vi "Keypad(subvi).vi"(6 "[ESC]":bool, 7 "DIO Ref Out 4":T1, 8 "error in (no error)":errorcluster, 9 "DIO Ref Out":T1, 10 "DIO Ref Out 2":T1, 11 "DIO Ref Out 3":T1) -> (0 "error out":errorcluster, 1 "Array":T8, 2 "Scan":bool[](array[boolean]), 3 "Index of current pressed button":i32)   [LabVIEW 2017]
uses:
  tranparent_key.ctl
  <vilib>/myRIO/Instrument Drivers/Onboard IO/DIO/typedefs/DIO Reference.ctl
  <vilib>/myRIO/Common/Instrument Driver Framework/Utilities/typedefs/myRIO Generic Hardware Reference.ctl
  <vilib>/myRIO/Common/Instrument Driver Framework/Utilities/typedefs/Hardware Version Enum.ctl
  <vilib>/myRIO/Common/Instrument Driver Framework/Utilities/typedefs/myRIO v1.0 Reference.ctl
  <vilib>/myRIO/Common/Instrument Driver Framework/Utilities/typedefs/Generic FPGA Reference.ctl
  <vilib>/myRIO/Common/Instrument Driver Framework/myRIO v1.0/DIO/typedefs/DIO Channels List.ctl
  <vilib>/myRIO/Common/Instrument Driver Framework/myRIO v1.0/DIO/typedefs/DIO Channels Enum.ctl
  <vilib>/Utility/error.llb/Error Cluster From Error Code.vi
  <vilib>/myRIO/Common/Instrument Driver Framework/myRIO v1.0/DIO/vis/myRIO v1.0 Read DIO.vi
  <vilib>/myRIO/Common/Instrument Driver Framework/myRIO v1.0/DIO/vis/myRIO v1.0 Write DIO.vi
  <vilib>/myRIO/Instrument Drivers/Onboard IO/DIO/vis/Smart Open.vi
  <vilib>/myRIO/Instrument Drivers/Onboard IO/DIO/DIO.lvlib
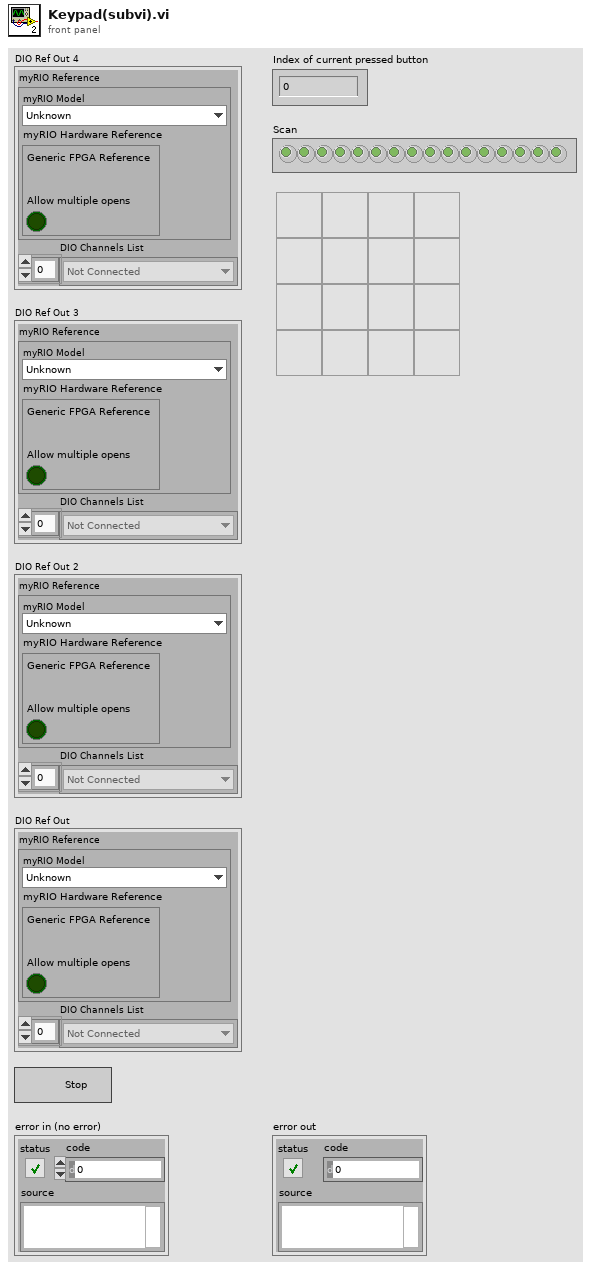
[diagram p1: front panel]
types:
  T1 = typedef "DIO.lvlib/DIO Reference.ctl" = cluster{"myRIO Reference":T2, "DIO Channels List":T6}
  T2 = typedef "myRIO Generic Hardware Reference.ctl" = cluster{"myRIO Model":T3, "myRIO Hardware Reference":T4}
  T3 = typedef "Hardware Version Enum.ctl" = enum16{"Unknown", "myRIO-1900", "myRIO-1950", "roboRIO", "NI ELVIS RIO CM"}
  T4 = typedef "myRIO v1.0 Reference.ctl" = cluster{"Generic FPGA Reference":T5, "Allow multiple opens":bool}
  T5 = typedef "Generic FPGA Reference.ctl" = refnum<k20>
  T6 = typedef "DIO Channels List.ctl" = T7[]
  T7 = typedef "DIO Channels Enum.ctl" = enum16{"Not Connected", "C/DIO0", "C/DIO1", "C/DIO2", "C/DIO3", "C/DIO4", "C/DIO5", "C/DIO6", "C/DIO7", "A/DIO0", "A/DIO1", "A/DIO2", "A/DIO3", "A/DIO4", "A/DIO5", "A/DIO6", "A/DIO7", "A/DIO8", "A/DIO9", "A/DIO10", "A/DIO11", "A/DIO12", "A/DIO13", "A/DIO14", "A/DIO15", "B/DIO0", "B/DIO1", "B/DIO2", "B/DIO3", "B/DIO4", "B/DIO5", "B/DIO6", "B/DIO7", "B/DIO8", "B/DIO9", "B/DIO10", "B/DIO11", "B/DIO12", "B/DIO13", "B/DIO14", "B/DIO15", "LED0", "LED1", "LED2", "LED3", "Button0", "DIO/DIO0", "DIO/DIO1", "DIO/DIO2", "DIO/DIO3", "DIO/DIO4", "DIO/DIO5", "DIO/DIO6", "DIO/DIO7", "DIO/DIO8", "DIO/DIO9", "SPI/CS0", "SPI/CS1", "SPI/CS2", "SPI/CS3", "LED RADIO (Green)", "LED RADIO (Red)", "LED COMM (Green)", "LED COMM (Red)", "LED MODE (Green)", "LED MODE (Red)"}
  T8 = typedef "tranparent_key.ctl" = bool[][]
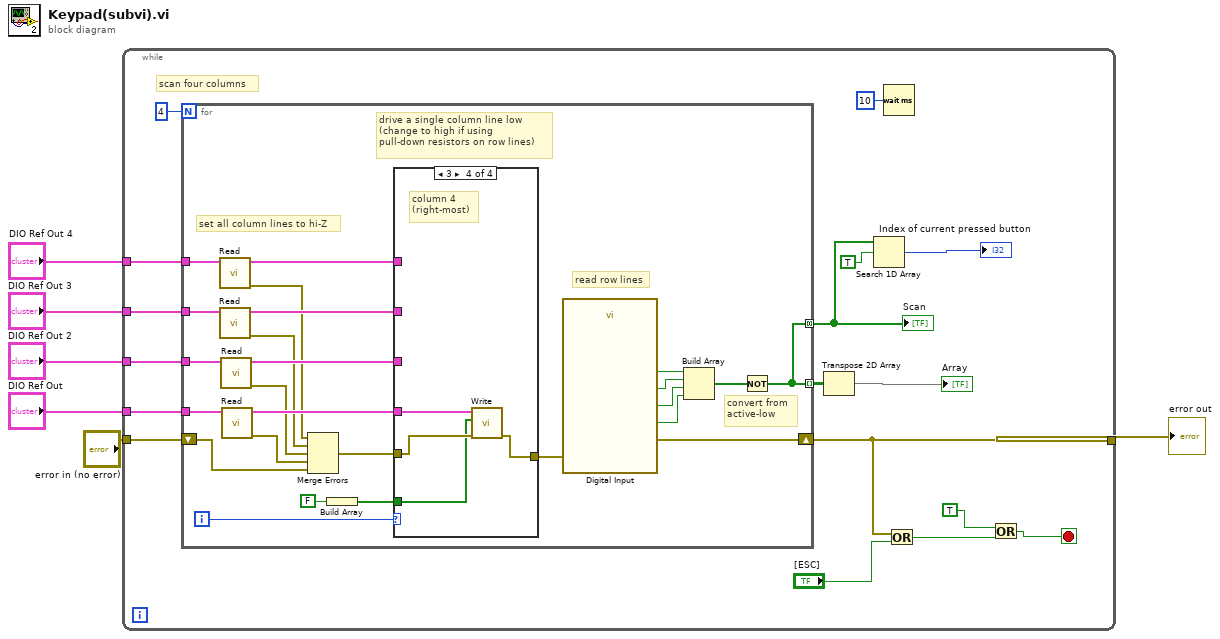
[diagram p0: block diagram]
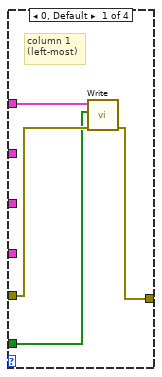
[diagram p2: hidden frame]
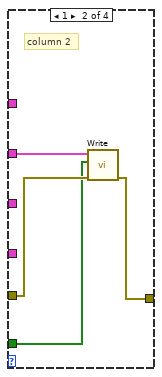
[diagram p3: hidden frame]
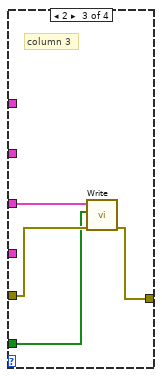
[diagram p4: hidden frame]
diagram:
  n1 = while {
    tunnel: [w20] -> w1
    tunnel: "DIO Ref Out 4" -> [w18]
    tunnel: "DIO Ref Out 3" -> [w17]
    tunnel: "DIO Ref Out 2" -> [w16]
    tunnel: "DIO Ref Out" -> [w15]
    tunnel: "error in (no error)" -> [w14]
    stop <- w7 stop-if-true
    # "scan four columns"
    n2 = for {
      N: 4 -> [_]
      tunnel: [w41] -> w19 mode=indexing
      shift-right: [w43] -> w20
      shift-left: w14 -> [w27]
      tunnel: [w41] -> w13 mode=concatenating
      tunnel: w18 -> [w40]
      tunnel: w17 -> [w37]
      tunnel: w16 -> [w38]
      tunnel: w15 -> [w39]
      i -> [w48]
      # "convert from\nactive-low"
      # "set all column lines to hi-Z"
      # "read row lines"
      # "drive a single column line low\n(change to high if using \npull-down resistors on row lines)"
      n3 = call <vilib>:"Read.vi"("DIO Ref In"=w40) -> ("error out"=w31:errorcluster, "DIO Ref Out"=w36:T1)  [unwired: 8 in, 1 out]
      n4 = call <vilib>:"Read.vi"("DIO Ref In"=w37) -> ("error out"=w30:errorcluster, "DIO Ref Out"=w35:T1)  [unwired: 8 in, 1 out]
      n5 = call <vilib>:"Read.vi"("DIO Ref In"=w38) -> ("error out"=w29:errorcluster, "DIO Ref Out"=w34:T1)  [unwired: 8 in, 1 out]
      n6 = call <vilib>:"Read.vi"("DIO Ref In"=w39) -> ("error out"=w28:errorcluster, "DIO Ref Out"=w33:T1)  [unwired: 8 in, 1 out]
      n7 = Merge Errors(w31, w30, w29, w28, w27) -> (w26:errorcluster)
      n8 = Build Array "Build Array"(FALSE) -> (w24:bool[])
      n9 = case shown="3" w48 {
        tunnel: w36 -> [w52 _ _ _]
        tunnel: w35 -> [_ w56 _ _]
        tunnel: w34 -> [_ _ w60 _]
        tunnel: w33 -> [_ _ _ w64]
        tunnel: [w51 w55 w59 w63] -> w32
        tunnel: w26 -> [w50 w54 w58 w62]
        tunnel: w24 -> [w49 w53 w57 w61]
        frame 0, Default {
          # "column 1\n(left-most)"
          n10 = call <vilib>:"Write.vi"("error in (no error)"=w50, "Values"=w49, "DIO Ref In"=w52) -> ("error out"=w51:errorcluster)  [unwired: 6 in, 1 out]
        }
        frame 1 {
          # "column 2"
          n11 = call <vilib>:"Write.vi"("error in (no error)"=w54, "Values"=w53, "DIO Ref In"=w56) -> ("error out"=w55:errorcluster)  [unwired: 6 in, 1 out]
        }
        frame 2 {
          # "column 3"
          n12 = call <vilib>:"Write.vi"("error in (no error)"=w58, "Values"=w57, "DIO Ref In"=w60) -> ("error out"=w59:errorcluster)  [unwired: 6 in, 1 out]
        }
        frame 3 {
          # "column 4\n(right-most)"
          n13 = call <vilib>:"Write.vi"("error in (no error)"=w62, "Values"=w61, "DIO Ref In"=w64) -> ("error out"=w63:errorcluster)  [unwired: 6 in, 1 out]
        }
      }
      n14 = call "Digital Input"("error in (no error)"=w32) -> ("B/DIO4 (Pin 19)"=w47:bool, "B/DIO5 (Pin 21)"=w46:bool, "B/DIO6 (Pin 23)"=w45:bool, "B/DIO7 (Pin 25)"=w44:bool, "error out"=w43:errorcluster)  [unwired: 22 in]
      n15 = Build Array "Build Array"(w47, w46, w45, w44) -> (w42:bool[])
      n16 = Not(x=w42) -> (.not. x?=w41:bool[])
    }
    "Scan" <- w13
    n17 = Transpose 2D Array(2D array=w19) -> (transposed array=→"Array":bool[][])
    n18 = Search 1D Array(1D array=w13, element=TRUE) -> (index of element=→"Index of current pressed button":i32)  [unwired: 1 in]
    n19 = Wait (ms)(milliseconds to wait=u32 10) -> ()  [unwired: 1 out]
    n20 = Or(x=w20, y="[ESC]") -> (x .or. y?=w8:bool)
    n21 = Or(x=TRUE, y=w8) -> (x .or. y?=w7:bool)
  }
  "error out" <- w1
